vi "Set SLSC Switch Topology.vi"(8 "error in":errorcluster, 10 "topology":string, 11 "slsc switch custom device in":T1 format="%.0x") -> (0 "error out":errorcluster, 3 "slsc switch custom device out":T1 format="%.0x")   [LabVIEW 2017, in "SLSC Switch Scripting.lvlib"]
uses:
  SLSC Switch Scripting.lvlib
  <vilib>/NI Veristand/Custom Device API/Custom Device Item Ref.ctl
  <vilib>/NI Veristand/Custom Device API/Custom Device API.lvlib
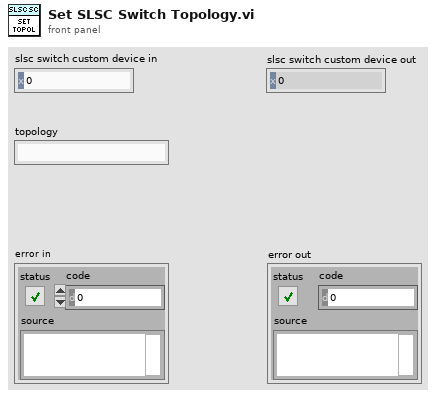
[diagram p1: front panel]
types:
  T1 = typedef "Custom Device API.lvlib/Custom Device Item Ref.ctl" = u64
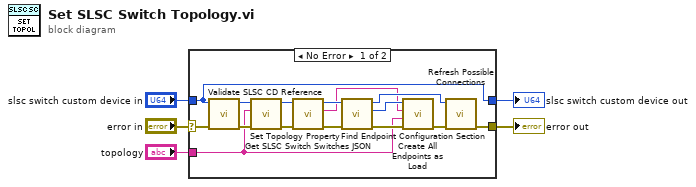
[diagram p0: block diagram]
diagram:
  n1 = case shown="No Error" "error in" {
    selector: "error in" -> [w7 w22]
    tunnel: "topology" -> [w6 _]
    tunnel: [w13 w22] -> w5
    tunnel: "slsc switch custom device in" -> [w8 w21]
    tunnel: [w8 w21] -> w2
    frame No Error {
      n2 = call "Validate SLSC CD Reference.vi"("error in (no error)"=w7, "SLSC Switch Custom Device Ref in"=w8) -> ("error out"=w9:errorcluster, "SLSC Switch Custom Device Ref out"=w10:T1)  [unwired: 8 in]
      n3 = call "Set Topology Property.vi"("error in (no error)"=w9, "Topology"=w6, "SLSC Switch Custom Device Ref in"=w10) -> ("error out"=w12:errorcluster, "SLSC Switch Custom Device Ref out"=w11:T1)  [unwired: 7 in]
      n4 = call "Get SLSC Switch Switches JSON.vi"("error in (no error)"=w12, "SLSC Switch Custom Device Ref in"=w11) -> ("error out"=w17:errorcluster, "Switches JSON"=w15:string, "SLSC Switch Custom Device Ref out"=w16:T1)  [unwired: 7 in]
      n5 = call "Find Endpoint Configuration Section.vi"("error in"=w17, "slsc switch custom device in"=w16) -> ("error out"=w18:errorcluster, "endpoint configuration"=w19:T1, "slsc switch custom device out"=w20:T1)  [unwired: 7 in]
      n6 = call "Create All Endpoints as Load.vi"("error in (no error)"=w18, "topology"=w6, "switches json"=w15, "Endpoint Config Section Ref"=w19) -> ("error out"=w14:errorcluster)  [unwired: 6 in, 1 out]
      n7 = call "Refresh Possible Connections.vi"("error in (no error)"=w14, "SLSC Switch Custom Device Ref in"=w20) -> ("error out"=w13:errorcluster)  [unwired: 8 in, 1 out]
    }
    frame Error {
    }
  }
  "error out" <- w5
  "slsc switch custom device out" <- w2
